vi "errorComp.vi"(10 "Error":T1, 11 "Position":T1) -> (3 "Compesated Position":T1)   [LabVIEW 2015]
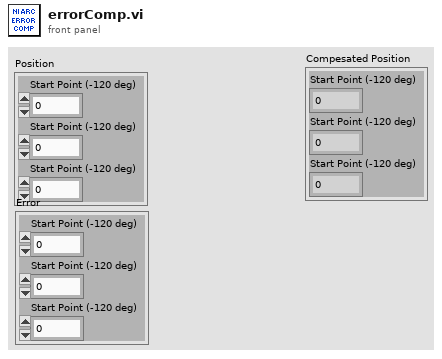
[diagram p1: front panel]
types:
  T1 = cluster{"Start Point (-120 deg)":dbl, "Start Point (-120 deg)":dbl, "Start Point (-120 deg)":dbl}
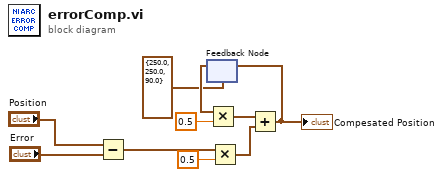
[diagram p0: block diagram]
diagram:
  n1 = Subtract(x="Position", y="Error") -> (x-y=w2:T1)
  n2 = feedback #1(T1 {"Start Point (-120 deg)"=250.0, "Start Point (-120 deg)"=250.0, "Start Point (-120 deg)"=90.0} ("Position 3")) -> (w9:T1)
  n3 = Multiply(x=w9, y=0.5) -> (x*y=w7:T1)
  n4 = Multiply(x=w2, y=0.5) -> (x*y=w6:T1)
  n5 = Add(x=w7, y=w6) -> (x+y=w1:T1)
  "Compesated Position" <- w1
  n6 = feedback-in #1(w1) -> ()
